vi "Tarea2.vi"() -> ()   [LabVIEW 2013]
panel:
  out "Sobresalientes":bool
  out "Muy buenos":bool
  out "Reprobados":bool
  out "Buenos":bool
  out "Sobresalientes":dbl
  out "Muy buenos":dbl
  out "Buenos":dbl
  out "Reprobados":dbl
  # "Generar la nota de 10 alumnos, luego ir contando cuantos alumnos estan en los siguientes rangos\n\n1-59 reprobados\n60-80 buenos\n81-90 muy buenos\n91-100 sobresalientes\n\nEncender un led para cada uno de los rangos."
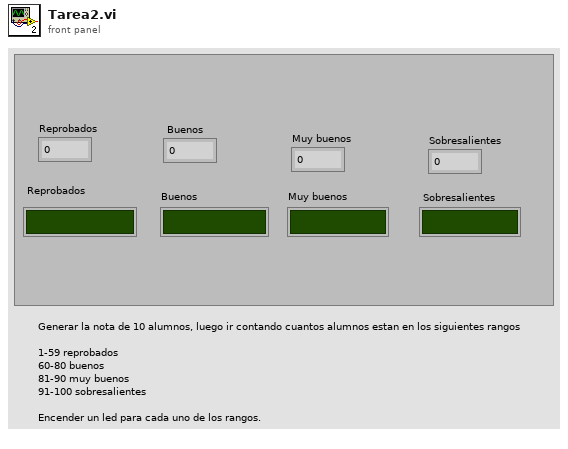
[diagram p1: front panel]
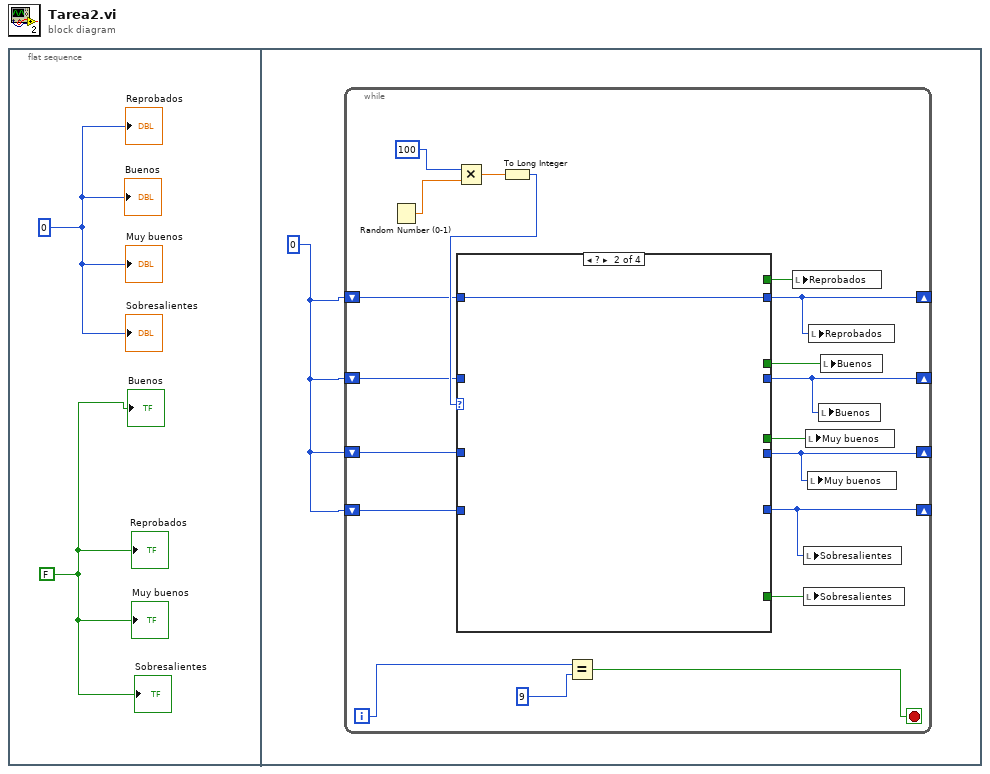
[diagram p0: block diagram]
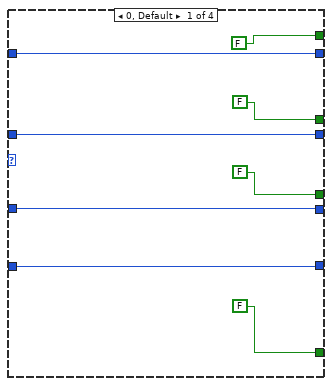
[diagram p2: hidden frame]
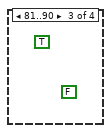
[diagram p3: hidden frame]
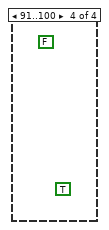
[diagram p4: hidden frame]
diagram:
  n1 = flat-sequence {
    frame #0 {
      w2 = FALSE
      w1 = 0
      "Reprobados" <- w1
      "Buenos" <- w1
      "Muy buenos" <- w1
      "Sobresalientes" <- w1
      "Buenos" <- w2
      "Reprobados" <- w2
      "Muy buenos" <- w2
      "Sobresalientes" <- w2
    }
    frame #1 {
      w3 = 0
      n2 = while {
        shift-right: [w14] -> _
        shift-left: w3 -> [w18]
        shift-right: [w13] -> _
        shift-left: w3 -> [w17]
        shift-right: [w12] -> _
        shift-left: w3 -> [w16]
        shift-right: [w11] -> _
        shift-left: w3 -> [w15]
        i -> [w5]
        stop <- w4 stop-if-true
        n3 = Random Number (0-1)() -> (number: 0 to 1=w21:dbl)
        n4 = Multiply(x=100, y=w21) -> (x*y=w20:dbl)
        n5 = To Long Integer(number=w20) -> (32bit integer=w19:i32)
        n6 = case w19 {
          tunnel: [w30 w31 _ _] -> w14
          tunnel: w18 -> [w30 w31 _ _]
          tunnel: w17 -> [w29 _ _ _]
          tunnel: [w29 _ _ _] -> w13
          tunnel: [w28 _ _ _] -> w12
          tunnel: w16 -> [w28 _ _ _]
          tunnel: w15 -> [w27 _ _ _]
          tunnel: [w27 _ _ _] -> w11
          tunnel: [FALSE _ _ _] -> w10
          tunnel: [FALSE _ _ _] -> w9
          tunnel: [FALSE _ _ _] -> w8
          tunnel: [FALSE _ _ _] -> w7
          frame 0, Default {
          }
          frame ? {
          }
          frame 81..90 {
            w32 = FALSE
            w33 = TRUE
          }
          frame 91..100 {
            w35 = FALSE
            w34 = TRUE
          }
        }
        n7 = Equal?(x=w5, y=9) -> (x = y?=w4:bool)
        n8 = local write "Reprobados"(w10) -> ()
        n9 = local write "Sobresalientes"(w11) -> ()
        n10 = local write "Sobresalientes"(w7) -> ()
        n11 = local write "Muy buenos"(w8) -> ()
        n12 = local write "Muy buenos"(w12) -> ()
        n13 = local write "Reprobados"(w14) -> ()
        n14 = local write "Buenos"(w13) -> ()
        n15 = local write "Buenos"(w9) -> ()
      }
    }
  }
